vi "HEWH RLT Delay Timer.vi"(8 "Error In":errorcluster, 10 "Delay After Cutout (sec)":dbl, 11 "Heat Source ON (1=ON)":bool) -> (0 "Error Out":errorcluster, 1 "Elapsed Time (sec)":dbl format="%.2f", 3 "Delay is Over":bool)   [LabVIEW 2019]
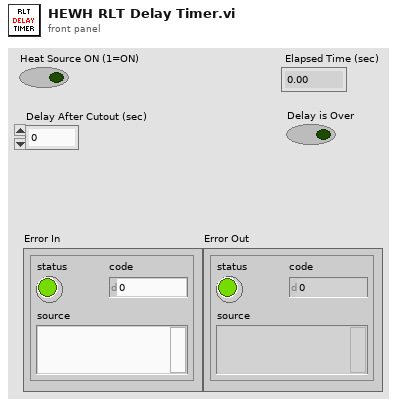
[diagram p1: front panel]
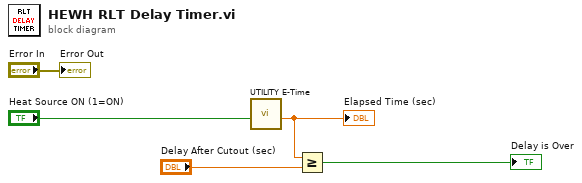
[diagram p0: block diagram]
diagram:
  n1 = call "UTILITY E-Time.vi"("Reset"="Heat Source ON (1=ON)") -> ("Elapsed Time (sec)"=w1:dbl)  [unwired: 8 in, 2 out]
  "Elapsed Time (sec)" <- w1
  n2 = Greater Or Equal?(x=w1, y="Delay After Cutout (sec)") -> (x >= y?=→"Delay is Over":bool)
  "Error Out" <- "Error In"
